vi "calculate axis ranges.vi"(8 "Iset Hist":dbl[](array[numeric]), 9 "Imon Hist":dbl[](array[numeric]), 10 "Vset Hist":dbl[](array[numeric]), 11 "Vmon Hist":dbl[](array[numeric])) -> (0 "Min I":dbl, 1 "Max I":dbl, 2 "Min V":dbl, 3 "Max V":dbl)   [LabVIEW 2018]
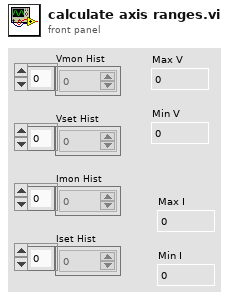
[diagram p1: front panel]
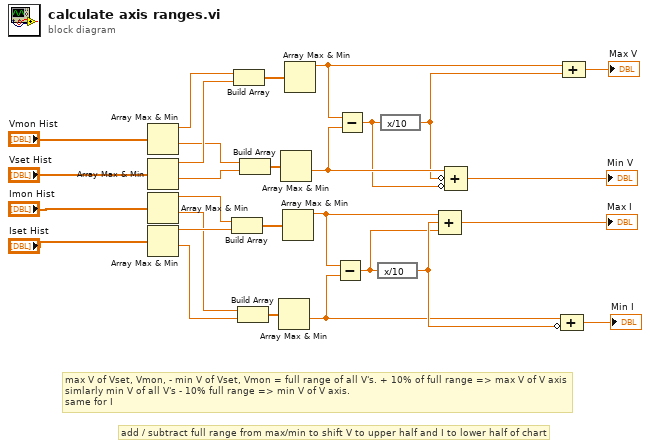
[diagram p0: block diagram]
diagram:
  # "add / subtract full range from max/min to shift V to upper half and I to lower half of chart"
  # "max V of Vset, Vmon, - min V of Vset, Vmon = full range of all V's. + 10% of full range => max V of V axis\nsimlarly min V of all V's - 10% full range => min V of V axis.\nsame for I"
  n1 = Array Max & Min(array="Vmon Hist") -> (max value=w23:dbl, min value=w20:dbl)  [unwired: 2 out]
  n2 = Array Max & Min(array="Vset Hist") -> (max value=w22:dbl, min value=w19:dbl)  [unwired: 2 out]
  n3 = Array Max & Min(array="Imon Hist") -> (max value=w6:dbl, min value=w4:dbl)  [unwired: 2 out]
  n4 = Array Max & Min(array="Iset Hist") -> (max value=w5:dbl, min value=w3:dbl)  [unwired: 2 out]
  n5 = Build Array(w6, w5) -> (w8:dbl[])
  n6 = Build Array(w23, w22) -> (w21:dbl[])
  n7 = Build Array(w4, w3) -> (w7:dbl[])
  n8 = Build Array(w20, w19) -> (w28:dbl[])
  n9 = Array Max & Min(array=w7) -> (min value=w12:dbl)  [unwired: 3 out]
  n10 = Array Max & Min(array=w28) -> (min value=w15:dbl)  [unwired: 3 out]
  n11 = Array Max & Min(array=w8) -> (max value=w9:dbl)  [unwired: 3 out]
  n12 = Array Max & Min(array=w21) -> (max value=w18:dbl)  [unwired: 3 out]
  n13 = Subtract(x=w9, y=w12) -> (x-y=w1:dbl)
  n14 = Subtract(x=w18, y=w15) -> (x-y=w2:dbl)
  n15 = expression code="x/10"(w1) -> (w13:dbl)
  n16 = expression code="x/10"(w2) -> (w14:dbl)
  n17 = Compound Arithmetic op=ADD(w9, w13, w1) -> (→"Max I":dbl)
  n18 = Compound Arithmetic op=ADD(w15, invert w14, invert w2) -> (→"Min V":dbl)
  n19 = Compound Arithmetic op=ADD(w12, invert w13) -> (→"Min I":dbl)
  n20 = Compound Arithmetic op=ADD(w18, w14) -> (→"Max V":dbl)
